vi "氨氮插入数据.vi"(0 "database":string, 1 "data":T1 {"单位" items=["ug/L", "mg/L", "ppm", "mg/m3", "cm", "ppb", "ug/m3", "%", "nmol/mol", "umol/mol", "MPN/L", "MPN/100ml", "ng/m3", "NTU", "无量纲", "ms/cm", "us/cm"]}, 3 "SN":string, 5 "table":string, 7 "测量模式":T2(ring)=enum."水样测试", 9 "数据标记表":string(combo)="N", 11 "error in (no error)":errorcluster) -> (15 "error out":errorcluster)   [LabVIEW 2016, in "斯坦道氨氮.lvlib"]
uses:
  <vilib>/Utility/sysdir.llb/System Directory Type.ctl
  <vilib>/Utility/error.llb/DialogType.ctl
  <vilib>/addons/database/Auxilliary.llb/DB Tools Transaction.ctl
  <vilib>/addons/database/Auxilliary.llb/DB Tools Isolation Level.ctl
  <vilib>/addons/database/Connection.llb/DB Tools Open Connec (String).vi
  <vilib>/addons/database/Connection.llb/Conn Execute.vi
  <vilib>/addons/database/Recordset.llb/Rec Destroy - Connection.vi
  <vilib>/addons/database/Recordset.llb/Rec Fetch Recordset Data (R).vi
  <vilib>/addons/database/Connection.llb/Conn Transaction.vi
  <vilib>/addons/database/NI_Database_API.lvlib
panel:
  out "为空？":bool
  out "recordset data":variant[][](array[variant])
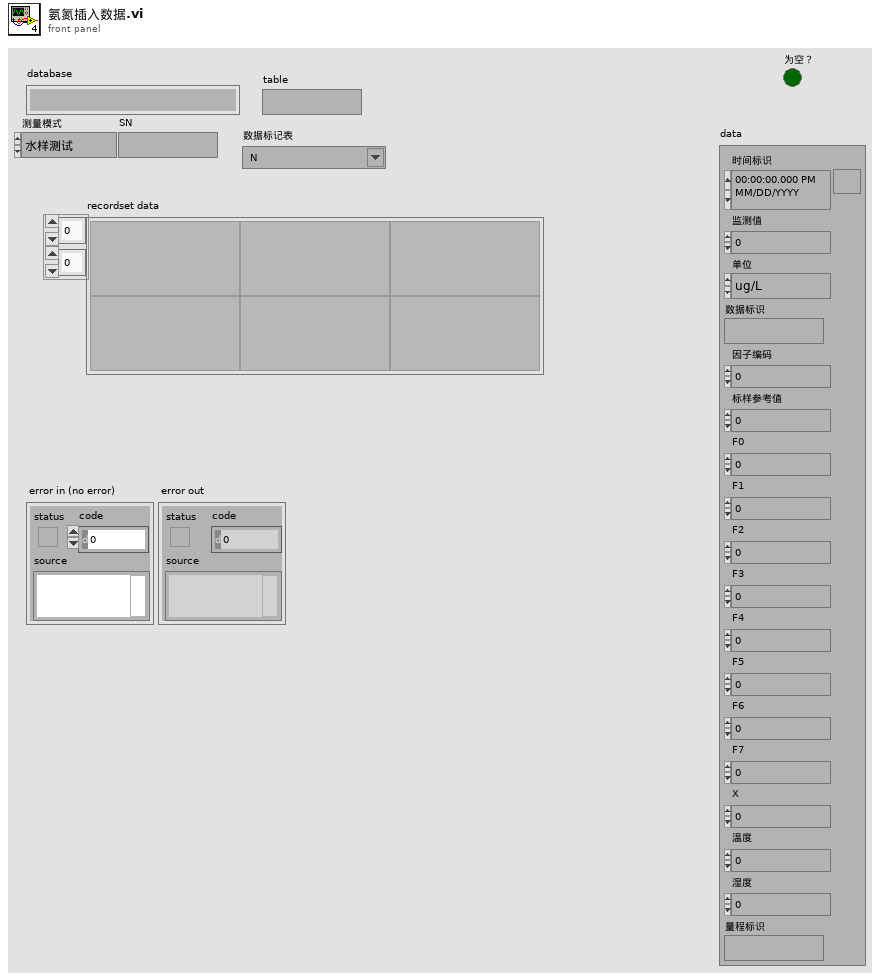
[diagram p1: front panel]
types:
  T1 = cluster{"时间标识":timestamp, "监测值":sgl, "单位":u16, "数据标识":string, "因子编码":u32, "标样参考值":sgl, "F0":sgl, "F1":sgl, "F2":sgl, "F3":sgl, "F4":sgl, "F5":sgl, "F6":sgl, "F7":sgl, "X":sgl, "温度":sgl, "湿度":sgl, "量程标识":string}
  T2 = enum16{"维护数据", "水样测试", "标样核查", "零点核查", "跨度核查", "空白测试", "平行样测试", "加标回收", "空白校准", "标样校准", "初始化（清洗）"}
  T3 = typedef "DialogType.ctl" = u16
  T4 = typedef "System Directory Type.ctl" = i32
  T5 = typedef "NI_Database_API.lvlib/Conn ObjectReference.ctl" = refnum<k1>
  T6 = typedef "NI_Database_API.lvlib/Rec ObjectReference.ctl" = refnum<k1>
  T7 = typedef "NI_Database_API.lvlib/DB Tools Transaction.ctl" = enum16{"begin", "commit", "rollback"}
  T8 = typedef "NI_Database_API.lvlib/DB Tools Isolation Level.ctl" = enum16{"chaos", "read uncommitted", "read committed", "repeatable read", "serializable"}
  T9 = cluster{"测量量程":dbl, "测量精度":dbl, "测量间隔":dbl, "消解温度":dbl, "消解时长":dbl, "空白校准时间":timestamp, "曲线截距":dbl, "曲线斜率":dbl, "测量检出限":dbl, "测量信号值":dbl, "线性相关系数":dbl, "二次多项式系数":dbl, "标样校准时间":timestamp, "稀释倍数":dbl, "三项式系数":dbl, "空白标定系数":dbl, "量程系数":dbl, "F0/ORPA":dbl, "F1/ORPB":dbl, "F2/ORPK":dbl, "F3":dbl, "F4":dbl, "F5":dbl, "F6":dbl, "F7":dbl, "X0/滴定数":dbl, "量程":dbl}
  T10 = cluster{"时间标识":timestamp, "测量模式":string, "数据类型":string, "监测值":sgl, "单位":string, "数据标识":string, "因子编码":string, "标样参考值":sgl, "F0":sgl, "F1":sgl, "F2":sgl, "F3":sgl, "F4":sgl, "F5":sgl, "F6":sgl, "F7":sgl, "X":sgl, "温度":sgl, "湿度":sgl, "量程标识":string, "SN":string, "Last Time":timestamp}
  T11 = cluster{"时间标识":timestamp, "设备":string, "日志信息":string}
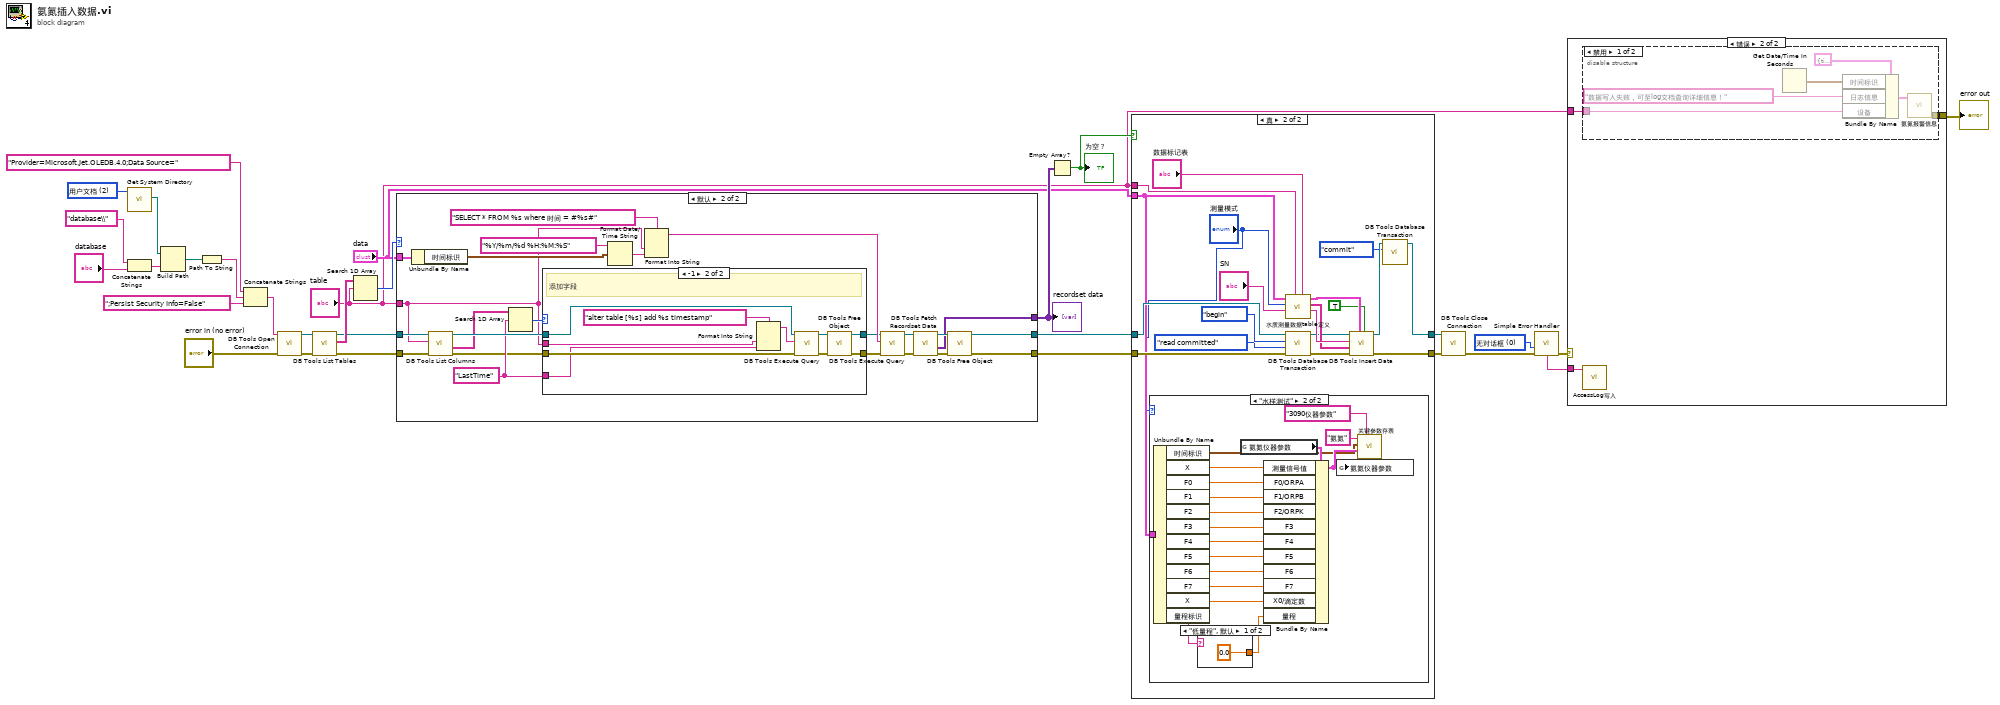
[diagram p0: block diagram]
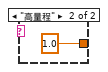
[diagram p6: hidden frame]
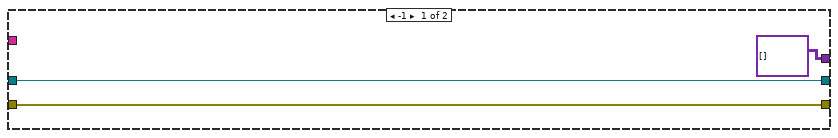
[diagram p7: hidden frame]
diagram:
  w5 = T3 0 items=["无对话框", "确定信息", "继续或停止信息", "确定信息＋警告", "继续/停止+警告"] ("type of dialog (OK msg:1)")
  w29 = T4 2 items=["用户目录"=0, "用户桌面"=1, "用户文档"=2, "用户应用程序数据"=3, "用户设置"=4, "用户临时目录"=5, "公共文档"=6, "公共应用程序数据"=7, "公共设置"=8, "公共缓存"=13, "系统核心库"=9, "系统安装库"=10, "应用程序文件"=11, "启动盘根目录"=12] ("system directory type")
  n1 = call <vilib>:"Get System Directory.vi"("system directory type"=w29) -> ("system directory"=w27:path)  [unwired: 10 in]
  n2 = Concatenate Strings("database\\" ("condition"), "database") -> (w21:string)
  n3 = Build Path(base path=w27, name or relative path=w21) -> (appended path=w26:path)
  n4 = Path To String(path=w26) -> (string=w25:string)
  n5 = Concatenate Strings("Provider=Microsoft.Jet.OLEDB.4.0;Data Source=" ("condition"), w25, ";Persist Security Info=False" ("condition")) -> (w23:string)
  n6 = call-poly <vilib>:"DB Tools Open Connection.vi"("error in (no error)"="error in (no error)", "connection information"=w23) -> ("error out"=w18:errorcluster, "connection reference"=w19:T5)  [unwired: 6 in]
  n7 = call <vilib>:"DB Tools List Tables.vi"("error in (no error)"=w18, "connection reference"=w19) -> ("error out"=w7:errorcluster, "tables"=w17:string[], "connection reference out"=w8:T5)  [unwired: 3 in]
  n8 = Search 1D Array(1D array=w17, element="table") -> (index of element=w16:i32)  [unwired: 1 in]
  n9 = case shown="默认" w16 {
    tunnel: [variant[][] [] ("recordset data") w52] -> w20
    tunnel: [w33 w51] -> w12
    tunnel: [w32 w50] -> w13
    tunnel: w8 -> [w33 w37]
    tunnel: w7 -> [w32 w36]
    tunnel: "table" -> [_ w35]
    tunnel: "data" -> [_ w45]
    frame -1 {
    }
    frame Default {
      w43 = "LastTime" ("元素")
      n10 = Unbundle By Name(w45) -> ("时间标识"=w48:timestamp)
      n11 = call <vilib>:"DB Tools List Columns.vi"("error in (no error)"=w36, "table"=w35, "connection reference"=w37) -> ("error out"=w41:errorcluster, "columns"=w42:string[], "connection reference out"=w44:T5)  [unwired: 1 in, 1 out]
      n12 = Search 1D Array(1D array=w42, element=w43) -> (index of element=w40:i32)  [unwired: 1 in]
      n13 = case shown="-1" w40 {
        tunnel: w44 -> [w58 w66]
        tunnel: w41 -> [w57 w65]
        tunnel: w43 -> [_ w63]
        tunnel: [w58 w61] -> w39
        tunnel: [w57 w60] -> w38
        tunnel: w35 -> [_ w59]
        frame 0, Default {
        }
        frame -1 {
          # "添加字段"
          n14 = Format Into String(format string="alter table [%s] add %s timestamp", w59, w63) -> (resulting string=w62:string)  [unwired: 2 in, 1 out]
          n15 = call-poly <vilib>:"DB Tools Execute Query.vi"("error in (no error)"=w65, "SQL query"=w62, "connection reference"=w66) -> ("error out"=w67:errorcluster, "recordset reference"=w68:T6)  [unwired: 5 in]
          n16 = call-poly <vilib>:"DB Tools Free Object.vi"("error in (no error)"=w67, "recordset reference"=w68) -> ("error out"=w60:errorcluster, "connection reference"=w61:T5)  [unwired: 8 in]
        }
      }
      n17 = Format Date/Time String(time format string (%c)="%Y/%m/%d %H:%M:%S" ("时间格式字符串(%c)"), seconds (now)=w48) -> (date/time string=w46:string)  [unwired: 1 in]
      n18 = Format Into String(format string="SELECT * FROM %s where 时间 = #%s#" ("格式字符串"), w35, w46) -> (resulting string=w49:string)  [unwired: 2 in, 1 out]
      n19 = call-poly <vilib>:"DB Tools Execute Query.vi"("error in (no error)"=w38, "SQL query"=w49, "connection reference"=w39) -> ("error out"=w53:errorcluster, "recordset reference"=w56:T6)  [unwired: 5 in]
      n20 = call-poly <vilib>:"DB Tools Fetch Recordset Data.vi"("error in (no error)"=w53, "recordset reference"=w56) -> ("error out"=w54:errorcluster, "recordset data"=w52:variant[][], "recordset reference out"=w55:T6)  [unwired: 3 in]
      n21 = call-poly <vilib>:"DB Tools Free Object.vi"("error in (no error)"=w54, "recordset reference"=w55) -> ("error out"=w50:errorcluster, "connection reference"=w51:T5)  [unwired: 8 in]
    }
  }
  "recordset data" <- w20
  n22 = Empty Array?(array=w20) -> (empty?=w14:bool)
  "为空？" <- w14
  n23 = case shown="真" w14 {
    tunnel: "table" -> [_ w89]
    tunnel: "data" -> [_ w72]
    tunnel: w13 -> [w69 w76]
    tunnel: w12 -> [w70 w88]
    tunnel: [w70 w78] -> w11
    tunnel: [w69 w82] -> w10
    frame False {
    }
    frame True {
      n24 = case shown="\"水样测试\"" "测量模式" {
        tunnel: w72 -> [_ w104]
        frame "维护数据", Default {
        }
        frame "水样测试" {
          n25 = Unbundle By Name(w104) -> ("时间标识"=w103:timestamp, "X"=w102:sgl, "F0"=w90:sgl, "F1"=w91:sgl, "F2"=w92:sgl, "F3"=w93:sgl, "F4"=w94:sgl, "F5"=w95:sgl, "F6"=w96:sgl, "F7"=w97:sgl, "X"=w98:sgl, "量程标识"=w100:string)
          n26 = case shown="\"低量程\", 默认" w100 {
            tunnel: [0.0 ("量程") 1.0 ("量程")] -> w99
            frame "低量程", Default {
            }
            frame "高量程" {
            }
          }
          n27 = global read "氨氮断电保存全局变量.vi" "氨氮仪器参数"() -> (w107:T9)
          n28 = Bundle By Name(cluster=w107, "测量信号值"=w102, "F0/ORPA"=w90, "F1/ORPB"=w91, "F2/ORPK"=w92, "F3"=w93, "F4"=w94, "F5"=w95, "F6"=w96, "F7"=w97, "X0/滴定数"=w98, "量程"=w99) -> (w105:T9)
          n29 = global write "氨氮断电保存全局变量.vi" "氨氮仪器参数"(w105) -> ()
          n30 = call "关键参数存表.vi"("table"="3090仪器参数", "仪器参数"=w105, "datatime"=w103, "仪器名称"="氨氮") -> ()  [unwired: 7 in, 1 out]
        }
      }
      n31 = call "水质测量数据table定义.vi"("数据标记表"="数据标记表", "table 输入"=w89, "SN"="SN", "测量模式"="测量模式", "data"=w72) -> ("table 输出"=w85:string, "columns"=w84:string[], "data输出"=w87:T10)  [unwired: 4 in]
      n32 = call-poly <vilib>:"DB Tools Database Transaction.vi"("error in (no error)"=w76, "isolation level (chaos)"=DB_Tools_Isolation_Level."read committed", "operation (begin)"=DB_Tools_Transaction."begin", "connection reference"=w88) -> ("error out"=w77:errorcluster, "connection reference out"=w79:T5)  [unwired: 2 in]
      n33 = call <vilib>:"DB Tools Insert Data.vi"("create table? (F)"=TRUE, "data"=w87, "error in (no error)"=w77, "columns"=w84, "table"=w85, "connection reference"=w79) -> ("error out"=w82:errorcluster, "connection reference out"=w83:T5)  [unwired: 4 in]
      n34 = call-poly <vilib>:"DB Tools Database Transaction.vi"("operation (begin)"=DB_Tools_Transaction."commit", "connection reference"=w83) -> ("connection reference out"=w78:T5)  [unwired: 4 in, 1 out]
    }
  }
  n35 = call <vilib>:"DB Tools Close Connection.vi"("error in (no error)"=w10, "connection reference"=w11) -> ("error out"=w6:errorcluster)  [unwired: 5 in]
  n36 = call <vilib>:"Simple Error Handler.vi"("type of dialog (OK msg:1)"=w5, "error in (no error)"=w6) -> ("error out"=w4:errorcluster, "message"=w3:string)  [unwired: 3 in, 3 out]
  n37 = case shown="错误" w4 {
    tunnel: w3 -> [_ w110]
    tunnel: [_ w112] -> w1
    tunnel: "table" -> [_ w111]
    frame No Error {
    }
    frame Error {
      n38 = call "AccessLog写入.vi"("Log"=w110) -> ()  [unwired: 11 in]
      n39 = disable-structure shown="禁用" {
        disable-tunnel: [w116 _] -> w112
        disable-tunnel: w111 -> [w114 _]
        frame Disabled {
          n40 = Get Date/Time In Seconds() -> (seconds since 1Jan1904=w115:timestamp)
          n41 = Bundle By Name(cluster=T11 {"时间标识"=timestamp(0 s since 1904-01-01), "设备"="", "日志信息"=""} ("data in"), "时间标识"=w115, "日志信息"="数据写入失败，可至log文档查询详细信息！", "设备"=w114) -> (w117:T11)
          n42 = call "氨氮报警信息.vi"("data in"=w117) -> ("error out"=w116:errorcluster)  [unwired: 10 in]
        }
        frame Enabled {
        }
      }
    }
  }
  "error out" <- w1
